vi "LaserFinding_Lines_v8.vi"(0 "Image In":T1, 3 "NoLaser":T1, 7 "error in":errorcluster) -> (20 "Image Out":T1, 21 "Straight Edge (Find Vert. Edge)":T2 {"Point2 (Real-World)"."Y" format="%.2f"; "Point2 (Real-World)"."X" format="%.2f"; "Point1 (Real-World)"."Y" format="%.2f"; "Point1 (Real-World)"."X" format="%.2f"; "Point2 (Pixels)"."Y" format="%.2f"; "Point2 (Pixels)"."X" format="%.2f"; "Point1 (Pixels)"."Y" format="%.2f"; "Point1 (Pixels)"."X" format="%.2f"}, 22 "Straight Edge (Find Horiz. Edge)":T2 {"Point2 (Real-World)"."Y" format="%.2f"; "Point2 (Real-World)"."X" format="%.2f"; "Point1 (Real-World)"."Y" format="%.2f"; "Point1 (Real-World)"."X" format="%.2f"; "Point2 (Pixels)"."Y" format="%.2f"; "Point2 (Pixels)"."X" format="%.2f"; "Point1 (Pixels)"."Y" format="%.2f"; "Point1 (Pixels)"."X" format="%.2f"}, 27 "error out":errorcluster)   [LabVIEW 2014]
uses:
  <vilib>/vision/Image Controls.llb/IMAQ Image.ctl
  <vilib>/vision/Measure.llb/Edge Options.ctl
  <vilib>/vision/Measure.llb/Edge Polarity.ctl
  <vilib>/vision/Measure.llb/Straight Edge Options.ctl
  <vilib>/vision/Measure.llb/Straight Edge Process.ctl
  <vilib>/vision/NI_Vision_Development_Module.lvlib
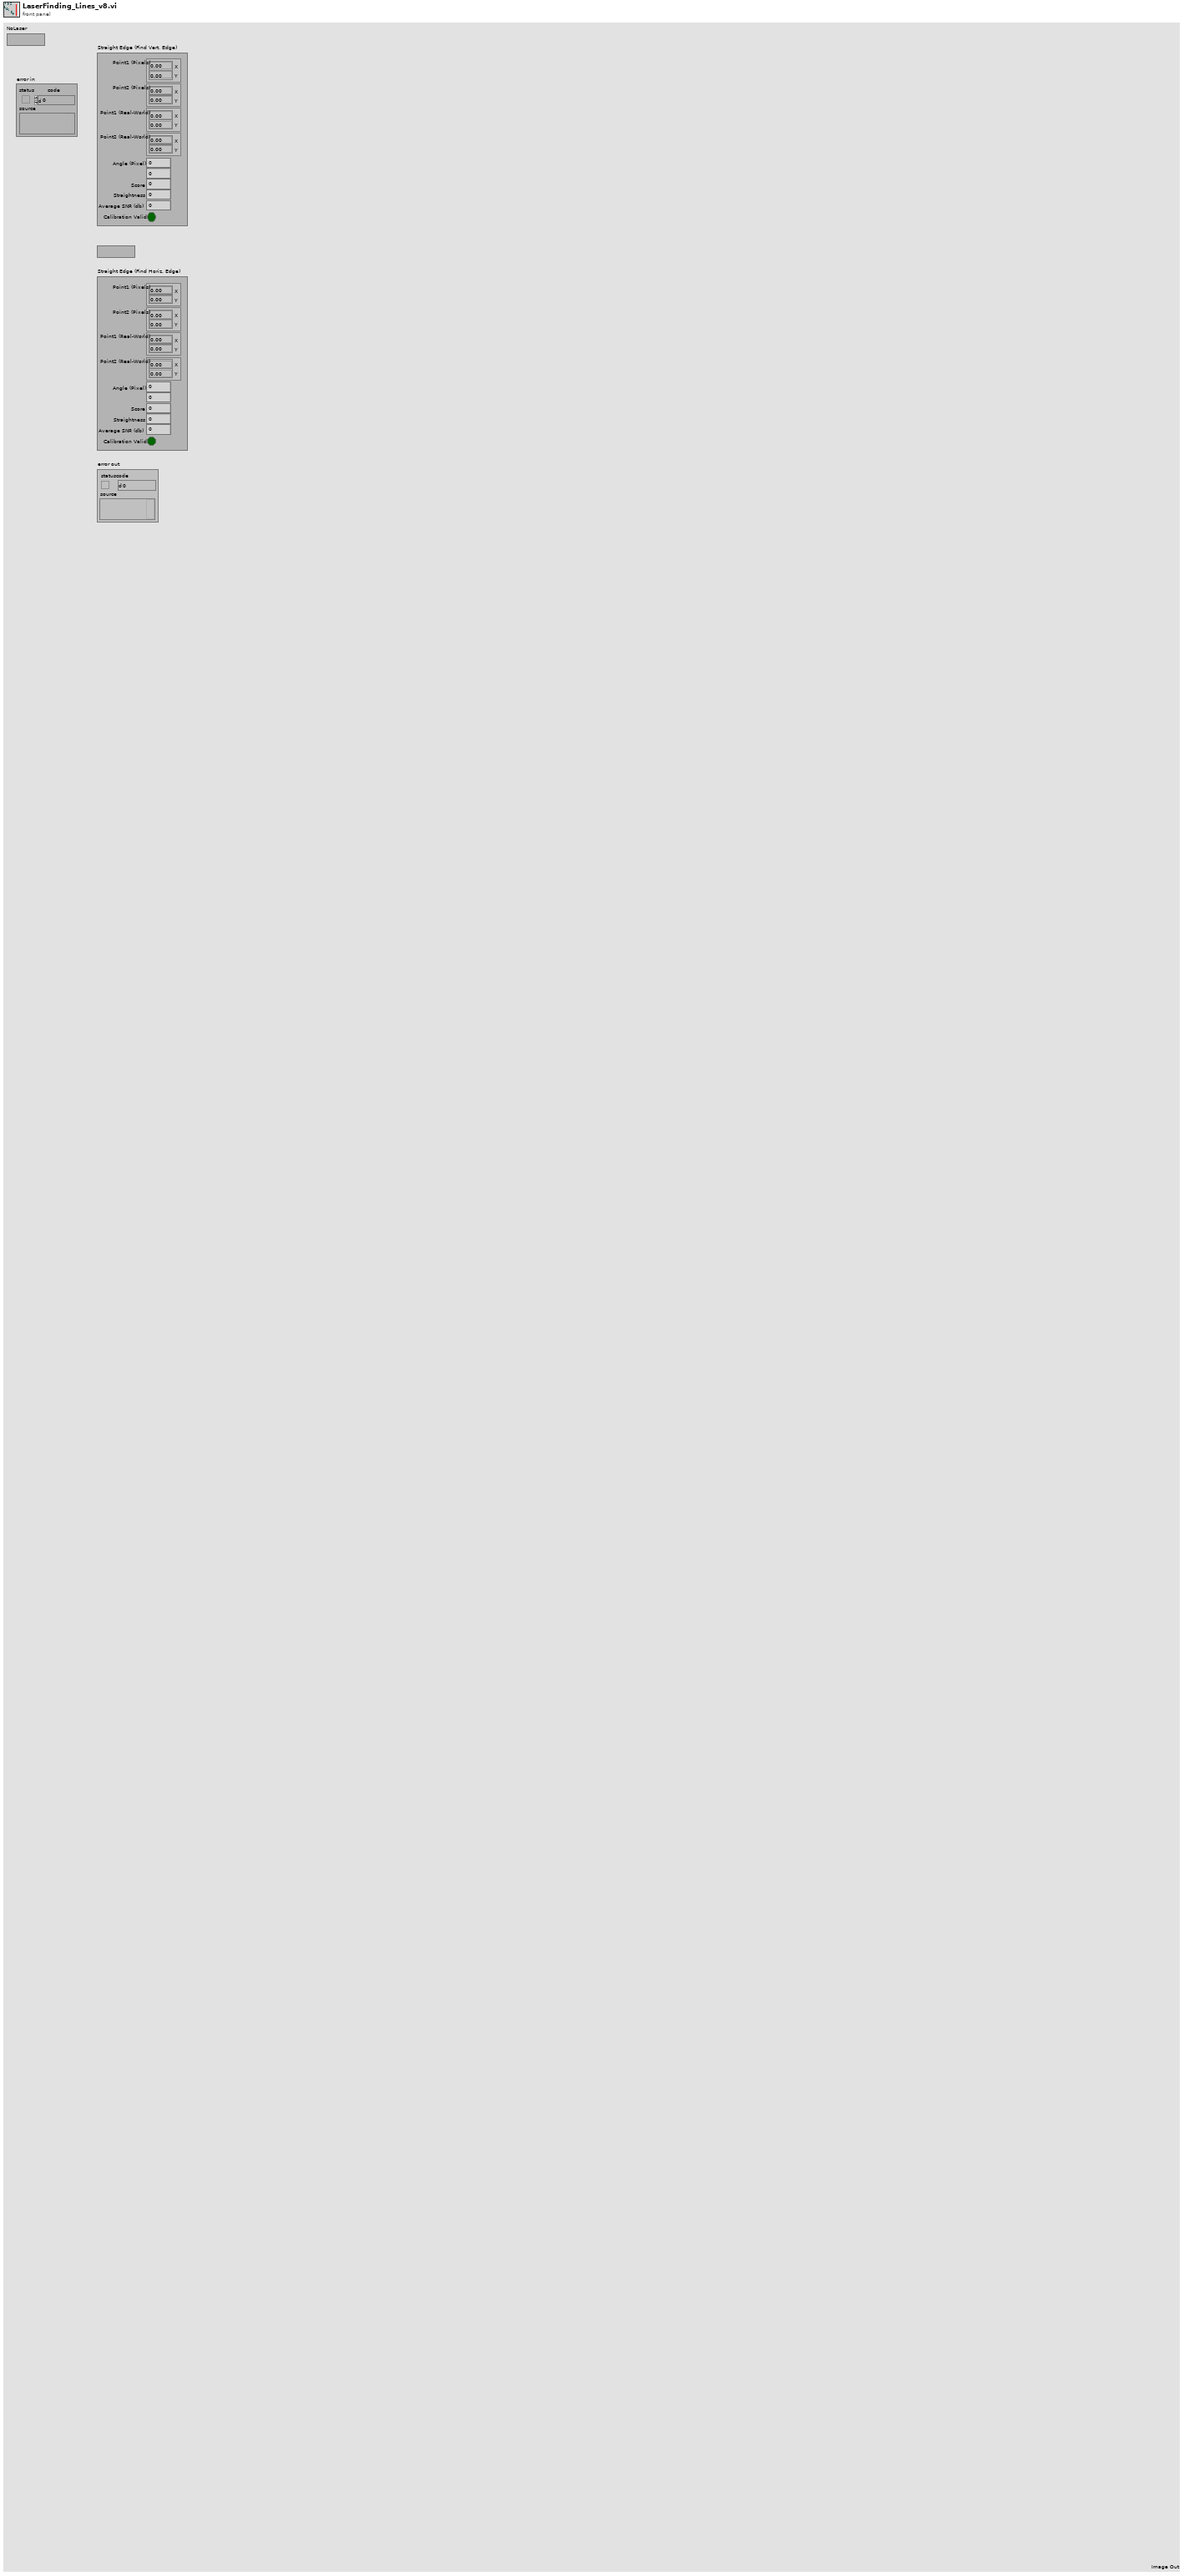
[diagram p1: front panel]
types:
  T1 = typedef "IMAQ Image.ctl" = refnum<image>
  T2 = cluster{"Point1 (Pixels)":cluster{"X":sgl, "Y":sgl}, "Point2 (Pixels)":cluster{"X":sgl, "Y":sgl}, "Point1 (Real-World)":cluster{"X":sgl, "Y":sgl}, "Point2 (Real-World)":cluster{"X":sgl, "Y":sgl}, "Angle (Pixel)":dbl, "Angle (Real-World)":dbl, "Score":dbl, "Straightness":dbl, "Average SNR (db)":dbl, "Calibration Valid":bool}
  T3 = typedef "Edge Options.ctl" = cluster{"Edge Polarity":T4, "Kernel Size":u32, "Width":u32, "Minimum Edge Strength":sgl, "Interpolation Type":enum32{"Zero Order", "Bilinear", "Quadratic", "Cubic", "Bilinear Fixed"}, "Data Processing Method":enum32{"Average", "Median"}}
  T4 = typedef "Edge Polarity.ctl" = u32
  T5 = cluster{"Search Direction":u32, "Edge Options":T3, "Show Search Area":bool, "Show Search Lines":bool, "Show Edges Found":bool, "Show Result":bool, "Search Area Color":u32, "Search Lines Color":u32, "Edge Locations Color":u32, "Result Color":u32, "Overlay Group Name":string}
  T6 = typedef "Straight Edge Options.ctl" = cluster{"Number of Lines":i32, "Type":T7, "Min. Score":dbl, "Max. Score":dbl, "Orientation":dbl, "Angle Range":dbl, "Angle Tolerance":dbl, "Step Size":u32, "Min. SNR (db)":dbl, "Min. Points (%)":dbl, "Hough Iterations":i32}
  T7 = typedef "Straight Edge Process.ctl" = enum32{"First Edge Rake", "Best Edge Rake", "Hough Edge Rake", "First Edge Projection", "Best Edge Projection"}
  T8 = cluster{"Global Rectangle":i32[], "Contours":cluster{"ID":enum32{"External", "Internal"}, "Type":u32, "Coordinates":i32[]}[]}
  T9 = cluster{"Measurement Parameter":i32, "Range Lower Value":dbl, "Range Upper Value":dbl, "Range":bool, "Measurement Type":bool}[]
  T10 = cluster{"histogram":u32[], "Minimal Value":sgl, "Maximal Value":sgl, "Starting Value":sgl, "Interval Width":sgl, "Mean Value":sgl, "Standard  Variation":sgl, "Area (pixels)":i32}
  T11 = typedef "Image Type" = u32
  T12 = cluster{"Point1 (Pixels)":cluster{"X":sgl, "Y":sgl}, "Point2 (Pixels)":cluster{"X":sgl, "Y":sgl}, "Point1 (Real-World)":cluster{"X":sgl, "Y":sgl}, "Point2 (Real-World)":cluster{"X":sgl, "Y":sgl}, "Angle (Pixel)":dbl, "Angle (Real-World)":dbl, "Score":dbl, "Straightness":dbl, "Average SNR (db)":dbl, "Calibration Valid":bool}[]
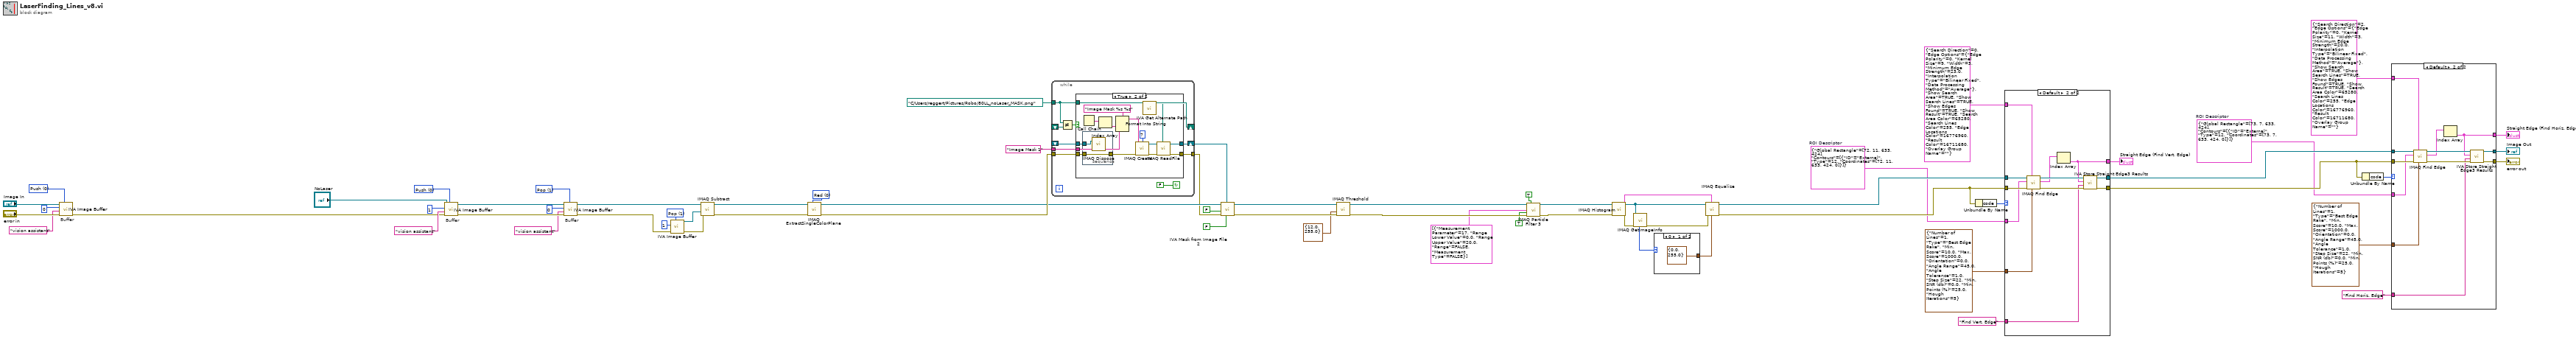
[diagram p0: block diagram]
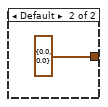
[diagram p4: hidden frame]
diagram:
  w9 = T8 {"Global Rectangle"=[73, 7, 633, 424], "Contours"=[{"ID"=enum."External", "Type"=12, "Coordinates"=[73, 7, 633, 424, 0]}]}  # ROI Descriptor
  w17 = T8 {"Global Rectangle"=[72, 11, 633, 424], "Contours"=[{"ID"=enum."External", "Type"=12, "Coordinates"=[72, 11, 633, 424, 0]}]}  # ROI Descriptor
  w44 = 0 items=["Red", "Green", "Blue", "Hue", "Saturation", "Luminance", "Value", "Intensity"] ("Color Plane")
  w50 = u16 1 items=["Push", "Pop", "Reset"] ("Function")
  w53 = u16 1 items=["Push", "Pop", "Reset"] ("Function")
  w58 = u16 0 items=["Push", "Pop", "Reset"] ("Function")
  w63 = u16 0 items=["Push", "Pop", "Reset"] ("Function")
  # "Buffer"
  # "Buffer"
  # "Buffer"
  n1 = call <vilib>:"IVA Image Buffer.vi"("Function"=w63, "error in (no error)"="error in", "Prefix"="vision assistant", "Buffer #"=0, "Image In"="Image In") -> ("error out"=w1:errorcluster)  [unwired: 6 out]
  n2 = call <vilib>:"IVA Image Buffer.vi"("Function"=w58, "error in (no error)"=w1, "Prefix"="vision assistant", "Buffer #"=1, "Image In"="NoLaser") -> ("error out"=w59:errorcluster, "Image Out"=w55:T1)  [unwired: 5 out]
  n3 = call <vilib>:"IVA Image Buffer.vi"("Function"=w53, "error in (no error)"=w59, "Prefix"="vision assistant", "Buffer #"=0, "Image In"=w55) -> ("error out"=w54:errorcluster, "Image Out"=w46:T1)  [unwired: 5 out]
  n4 = call <vilib>:"IVA Image Buffer.vi"("Function"=w50, "error in (no error)"=w54, "Buffer #"=1) -> ("error out"=w47:errorcluster, "Image Out"=w48:T1)  [unwired: 2 in, 5 out]
  n5 = call "IMAQ Subtract"("Image Src A"=w46, "Image Src B"=w48, "error in (no error)"=w47) -> ("Image Dst Out"=w43:T1, "error out"=w45:errorcluster)  [unwired: 2 in, 2 out]
  n6 = call "IMAQ ExtractSingleColorPlane"("Color Plane"=w44, "error in (no error)"=w45, "Image Src"=w43) -> ("error out"=w42:errorcluster, "Image Dst Out"=w39:T1)  [unwired: 1 in, 6 out]
  n7 = while {
    shift-right: [w74] -> w35
    shift-left: _ -> [w73]
    tunnel: [w71] -> w36
    tunnel: w42 -> [w70]
    tunnel: path "C:/Users/reggert/Pictures/Robo/80LL_noLaser_MASK.png" ("FilePath") -> [w66]
    tunnel: "Image Mask 1" ("Step Name") -> [w69]
    shift-right: [w66] -> _
    shift-left: _ -> [w68]
    stop <- FALSE continue-if-true
    n8 = Not Equal?(x=w66, y=w68) -> (x != y?=w67:bool)
    n9 = case shown="True" w67 {
      tunnel: [w76 w88] -> w74
      tunnel: w73 -> [w76 w80]
      tunnel: [w75 w86] -> w71
      tunnel: w70 -> [w75 w81]
      tunnel: w66 -> [_ w78]
      tunnel: w69 -> [_ w82]
      frame False {
      }
      frame True {
        n10 = Call Chain() -> (call chain=w84:string[])
        n11 = stacked-sequence {
          tunnel: w81 -> [w92]
          tunnel: w80 -> [w93]
          tunnel: [w92] -> w79
          frame #0 {
            n12 = call "IMAQ Dispose"("Image"=w93) -> ()  [unwired: 2 in, 4 out]
          }
        }
        n13 = Index Array(array=w84) -> (element=w83:string)  [unwired: 1 in]
        n14 = Format Into String(format string="Image Mask %s %s" ("Image Name"), w83, w82) -> (resulting string=w91:string)  [unwired: 2 in, 1 out]
        n15 = call "IMAQ Create"("Border Size"=7, "Image Name"=w91, "error in (no error)"=w79) -> ("New Image"=w89:T1, "error out"=w87:errorcluster)  [unwired: 1 in, 1 out]
        n16 = call <vilib>:"IVA Get Alternate Path.vi"("Path In"=w78) -> ("Path Out"=w77:path)  [unwired: 10 out]
        n17 = call "IMAQ ReadFile"("File Path"=w77, "error in (no error)"=w87, "Image"=w89) -> ("error out"=w86:errorcluster, "Image Out"=w88:T1)  [unwired: 2 in, 5 out]
      }
    }
  }
  n18 = call <vilib>:"IVA Mask from Image File 2.vi"("Shrink"=FALSE, "Image Mask"=w35, "error in (no error)"=w36, "Out / In"=FALSE, "Image Src"=w39) -> ("error out"=w38:errorcluster, "Image Out"=w32:T1)  [unwired: 1 in, 4 out]
  n19 = call "IMAQ Threshold"("error in (no error)"=w38, "Range"=cluster{"Lower value":sgl, "Upper value":sgl} {"Lower value"=12.0, "Upper value"=255.0}, "Image Src"=w32) -> ("error out"=w31:errorcluster, "Image Dst Out"=w27:T1)  [unwired: 3 in, 4 out]
  n20 = call "IMAQ Particle Filter 3"("Image Src"=w27, "Connectivity 4/8 (8)"=TRUE, "Selection Values"=T9 [{"Measurement Parameter"=17, "Range Lower Value"=0.0, "Range Upper Value"=20.0, "Range"=FALSE, "Measurement Type"=FALSE}], "Keep/Remove Particles (F)"=TRUE ("Keep/Remove Particles"), "error in (no error)"=w31) -> ("Image Dst Out"=w22:T1, "error out"=w28:errorcluster)  [unwired: 4 in, 5 out]
  n21 = call "IMAQ Histogram"("error in (no error)"=w28, "Image"=w22) -> ("error out"=w21:errorcluster, "Histogram Report"=w24:T10)  [unwired: 3 in, 5 out]
  n22 = call "IMAQ GetImageInfo"("error in (no error)"=w21, "Image"=w22) -> ("error out"=w20:errorcluster, "Image Type"=w23:T11)  [unwired: 8 out]
  n23 = case shown="0" w23 {
    tunnel: [cluster{"Minimum":sgl, "Maximum":sgl} {"Minimum"=0.0, "Maximum"=255.0} ("Range") cluster{"Minimum":sgl, "Maximum":sgl} {"Minimum"=0.0, "Maximum"=0.0} ("Range")] -> w19
    frame 0 {
    }
    frame Default {
    }
  }
  n24 = call "IMAQ Equalize"("Range"=w19, "Histogram Report"=w24, "error in (no error)"=w20, "Image Src"=w22) -> ("error out"=w25:errorcluster, "Image Dst Out"=w18:T1)  [unwired: 2 in, 4 out]
  n25 = Unbundle By Name(w25) -> ("code"=w14:i32)
  n26 = case shown="Default" w14 {
    tunnel: w18 -> [w96 w108]
    tunnel: w25 -> [_ w107]
    tunnel: w17 -> [_ w101]
    tunnel: [w96 w105] -> w10
    tunnel: [_ w103] -> w16
    tunnel: "Find Vert. Edge" ("Step Name") -> [_ w102]
    tunnel: T6 {"Number of Lines"=1, "Type"=enum."Best Edge Rake", "Min. Score"=10.0, "Max. Score"=1000.0, "Orientation"=0.0, "Angle Range"=45.0, "Angle Tolerance"=1.0, "Step Size"=22, "Min. SNR (db)"=0.0, "Min. Points (%)"=25.0, "Hough Iterations"=5} ("Fit Options") -> [_ w100]
    tunnel: T5 {"Search Direction"=0, "Edge Options"={"Edge Polarity"=0, "Kernel Size"=9, "Width"=3, "Minimum Edge Strength"=23.0, "Interpolation Type"=enum."Bilinear Fixed", "Data Processing Method"=enum."Average"}, "Show Search Area"=TRUE, "Show Search Lines"=TRUE, "Show Edges Found"=TRUE, "Show Result"=TRUE, "Search Area Color"=65280, "Search Lines Color"=255, "Edge Locations Color"=16776960, "Result Color"=16711680, "Overlay Group Name"=""} ("Options") -> [_ w99]
    tunnel: [_ w97] -> w11
    frame -1074396199, -1074396198 {
      # "Discard Coordinate System Error"
    }
    frame Default {
      n27 = call "IMAQ Find Edge"("Line Fit Options"=w100, "Options"=w99, "error in (no error)"=w107, "ROI Descriptor"=w101, "Image"=w108) -> ("error out"=w104:errorcluster, "Straight Edges"=w98:T12, "Image Out"=w106:T1)  [unwired: 1 in, 3 out]
      n28 = Index Array(array=w98) -> (element=w97:T2)  [unwired: 1 in]
      n29 = call <vilib>:"IVA Store Straight Edge3 Results.vi"("error in (no error)"=w104, "Step Name"=w102, "Straight Edge"=w97, "Image in"=w106) -> ("error out"=w103:errorcluster, "Image dup"=w105:T1)  [unwired: 1 in, 5 out]
    }
  }
  "Straight Edge (Find Vert. Edge)" <- w11
  n30 = Unbundle By Name(w16) -> ("code"=w5:i32)
  n31 = case shown="Default" w5 {
    tunnel: w10 -> [w109 w121]
    tunnel: w16 -> [_ w120]
    tunnel: w9 -> [_ w114]
    tunnel: [w109 w118] -> w8
    tunnel: [_ w116] -> w7
    tunnel: "Find Horiz. Edge" ("Step Name") -> [_ w115]
    tunnel: T6 {"Number of Lines"=1, "Type"=enum."Best Edge Rake", "Min. Score"=10.0, "Max. Score"=1000.0, "Orientation"=0.0, "Angle Range"=45.0, "Angle Tolerance"=1.0, "Step Size"=22, "Min. SNR (db)"=0.0, "Min. Points (%)"=25.0, "Hough Iterations"=5} ("Fit Options") -> [_ w113]
    tunnel: T5 {"Search Direction"=2, "Edge Options"={"Edge Polarity"=0, "Kernel Size"=11, "Width"=3, "Minimum Edge Strength"=20.0, "Interpolation Type"=enum."Bilinear Fixed", "Data Processing Method"=enum."Average"}, "Show Search Area"=TRUE, "Show Search Lines"=TRUE, "Show Edges Found"=TRUE, "Show Result"=TRUE, "Search Area Color"=65280, "Search Lines Color"=255, "Edge Locations Color"=16776960, "Result Color"=16711680, "Overlay Group Name"=""} ("Options") -> [_ w112]
    tunnel: [_ w110] -> w2
    frame -1074396199, -1074396198 {
      # "Discard Coordinate System Error"
    }
    frame Default {
      n32 = call "IMAQ Find Edge"("Line Fit Options"=w113, "Options"=w112, "error in (no error)"=w120, "ROI Descriptor"=w114, "Image"=w121) -> ("error out"=w117:errorcluster, "Straight Edges"=w111:T12, "Image Out"=w119:T1)  [unwired: 1 in, 3 out]
      n33 = Index Array(array=w111) -> (element=w110:T2)  [unwired: 1 in]
      n34 = call <vilib>:"IVA Store Straight Edge3 Results.vi"("error in (no error)"=w117, "Step Name"=w115, "Straight Edge"=w110, "Image in"=w119) -> ("error out"=w116:errorcluster, "Image dup"=w118:T1)  [unwired: 1 in, 5 out]
    }
  }
  "Image Out" <- w8
  "error out" <- w7
  "Straight Edge (Find Horiz. Edge)" <- w2
